vi "Lock-Unlock Front Panel.vi"(8 "error in (no error)":errorcluster, 10 "Lock?":bool, 11 "VISA resource name":refnum<visa-resource-name>) -> (0 "error out":errorcluster, 2 "Panel Locked?":bool, 3 "VISA resource name out":refnum<visa-resource-name>)   [LabVIEW 2018, in "DPO4104.lvlib" / "DPO4104.lvclass"]
doc: "This VI sends command for locking or unlocking the oscilloscope front panel."
uses:
  DPO4104.lvclass
  <instrlib>/Tektronix DPO MSO 2000 4000 Series/Tektronix DPO MSO 2000 4000 Series.lvlib
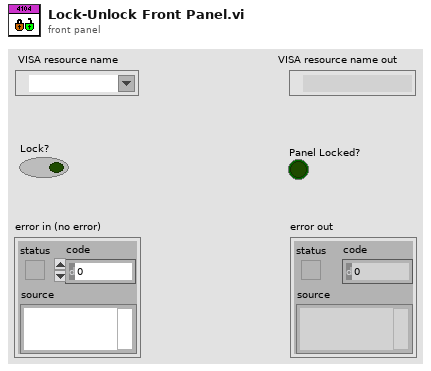
[diagram p1: front panel]
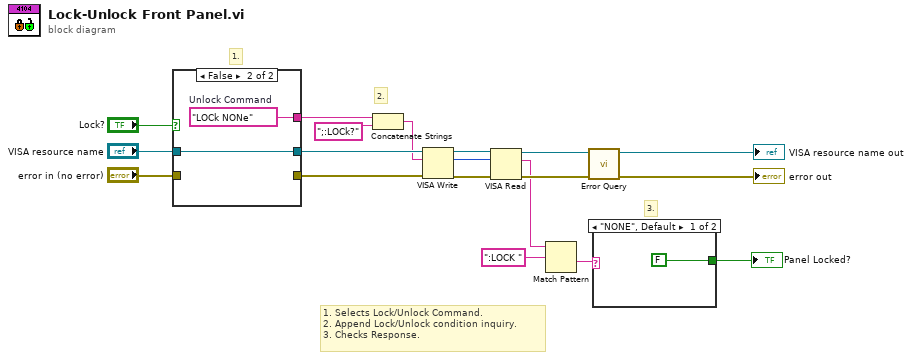
[diagram p0: block diagram]
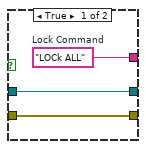
[diagram p2: hidden frame]
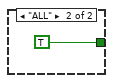
[diagram p3: hidden frame]
diagram:
  # "3."
  # "2."
  # "1."
  # "1. Selects Lock/Unlock Command.\n2. Append Lock/Unlock condition inquiry.\n3. Checks Response."
  n1 = case shown="False" "Lock?" {
    tunnel: [w22 w24] -> w3
    tunnel: [w21 _] -> w9
    tunnel: "error in (no error)" -> [w21 _]
    tunnel: "VISA resource name" -> [w20 w23]
    tunnel: [w20 w23] -> w7
    frame True {
      w22 = "LOCk ALL"  # Lock Command
    }
    frame False {
      w24 = "LOCk NONe"  # Unlock Command
    }
  }
  n2 = Concatenate Strings(w3, ";:LOCk?") -> (w1:string)
  n3 = VISA Write(VISA resource name=w7, write buffer=w1, error in (no error)=w9) -> (VISA resource name out=w6:refnum<visa-resource-name>, return count=w4:u32, error out=w5:errorcluster)
  n4 = VISA Read(VISA resource name=w6, byte count=w4, error in (no error)=w5) -> (VISA resource name out=w16:refnum<visa-resource-name>, read buffer=w15:string, error out=w17:errorcluster)  [unwired: 1 out]
  n5 = Match Pattern(string=w15, regular expression=":LOCK ") -> (after substring=w13:string)  [unwired: 1 in, 3 out]
  n6 = call <instrlib>:"Error Query.vi"("error in (no error)"=w17, "VISA resource name"=w16) -> ("error out"=→"error out":errorcluster, "VISA resource name out"=→"VISA resource name out":refnum<visa-resource-name>)  [unwired: 6 in, 2 out]
  n7 = case shown="\"NONE\", Default" w13 {
    tunnel: [FALSE TRUE] -> w12
    frame "NONE", Default {
    }
    frame "ALL" {
    }
  }
  "Panel Locked?" <- w12
